vi "resize_image_to_display.vi"(10 "DrawAreaSize":T1, 11 "image data":T2) -> (2 "Zoom factor":dbl)   [LabVIEW 2022 SP3]
doc: "Resize image by creating new Zoom factor, based on image window size (DrawAreaSize) and image size (from image data), which can be passed to picture's property node."
uses:
  <vilib>/picture/picture.llb/imagedata.ctl
  <vilib>/Utility/miscctls.llb/LVBoundsTypeDef.ctl
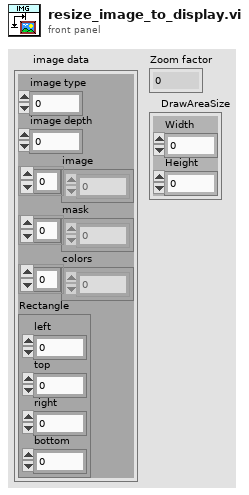
[diagram p1: front panel]
types:
  T1 = typedef "LVBoundsTypeDef.ctl" = cluster{"Width":u32, "Height":u32}
  T2 = typedef "imagedata.ctl" = cluster{"image type":i32, "image depth":i32, "image":u8[], "mask":u8[], "colors":u32[], "Rectangle":cluster{"left":i16, "top":i16, "right":i16, "bottom":i16}}
  T3 = cluster{"left":i16, "top":i16, "right":i16, "bottom":i16}
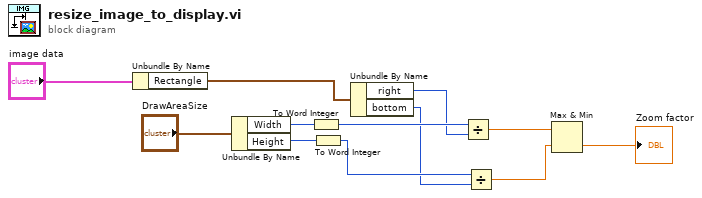
[diagram p0: block diagram]
diagram:
  n1 = Unbundle By Name("image data") -> ("Rectangle"=w8:T3)
  n2 = Unbundle By Name("DrawAreaSize") -> ("Width"=w12:u32, "Height"=w11:u32)
  n3 = To Word Integer(number=w12) -> (16bit integer=w10:i16)
  n4 = To Word Integer(number=w11) -> (16bit integer=w9:i16)
  n5 = Unbundle By Name(w8) -> ("right"=w7:i16, "bottom"=w6:i16)
  n6 = Divide(x=w10, y=w7) -> (x/y=w5:dbl)
  n7 = Divide(x=w9, y=w6) -> (x/y=w4:dbl)
  n8 = Max & Min(x=w5, y=w4) -> (min(x,y)=→"Zoom factor":dbl)  [unwired: 1 out]
